vi "notify_subvi.vi"() -> ()   [LabVIEW 2023]
panel:
  out "latest notification":dbl[](array[numeric])
  in  "Stop Button":bool
  in  "Array":dbl[](array[numeric])
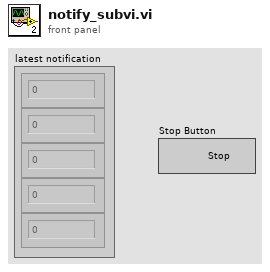
[diagram p1: front panel]
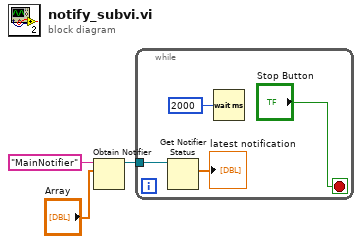
[diagram p0: block diagram]
diagram:
  n1 = Obtain Notifier(name (unnamed)="MainNotifier", notification data type="Array") -> (notifier out=w1:refnum<notifier>)  [unwired: 2 in, 2 out]
  n2 = while {
    tunnel: w1 -> [w6]
    stop <- "Stop Button" stop-if-true
    n3 = Get Notifier Status(notifier=w6) -> (current notification=→"latest notification":dbl[])  [unwired: 1 in, 4 out]
    n4 = Wait (ms)(milliseconds to wait=u32 2000) -> ()  [unwired: 1 out]
  }
